vi "LuxResistance.vi"(1 "Vout":dbl) -> (0 "Resistance (kOhms)":dbl)   [LabVIEW 2021]
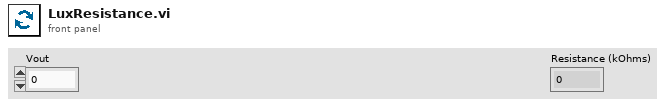
[diagram p1: front panel]
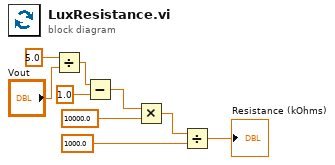
[diagram p0: block diagram]
diagram:
  n1 = Divide(x=5.0, y="Vout") -> (x/y=w6:dbl)
  n2 = Subtract(x=w6, y=1.0) -> (x-y=w4:dbl)
  n3 = Multiply(x=w4, y=10000.0) -> (x*y=w2:dbl)
  n4 = Divide(x=w2, y=1000.0) -> (x/y=→"Resistance (kOhms)":dbl)
